vi "test_Import Configuration_Error.vi"(8 "error in (no error)":errorcluster, 11 "TestCase in":refnum<class "FPGA Addon Scripting API Unit Tests.lvclass">=refnum) -> (0 "error out":errorcluster, 3 "TestCase out":refnum<class "FPGA Addon Scripting API Unit Tests.lvclass">)   [LabVIEW 2026, in "FPGA Addon Scripting API Unit Tests.lvclass"]
uses:
  FPGA Addon Scripting API Unit Tests.lvclass
  FPGA Addon Test Class/FPGA Addon Test Class.lvclass
  APIs/Scripting API/Scripting API.lvlib
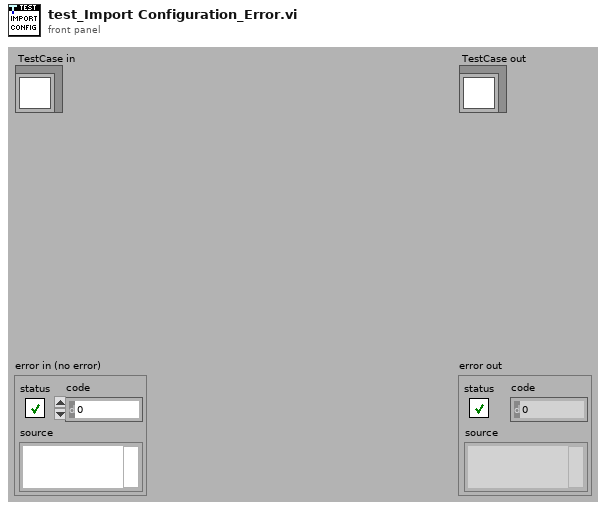
[diagram p1: front panel]
types:
  T1 = typedef "Custom Device API.lvlib/Custom Device Item Ref.ctl" = u64
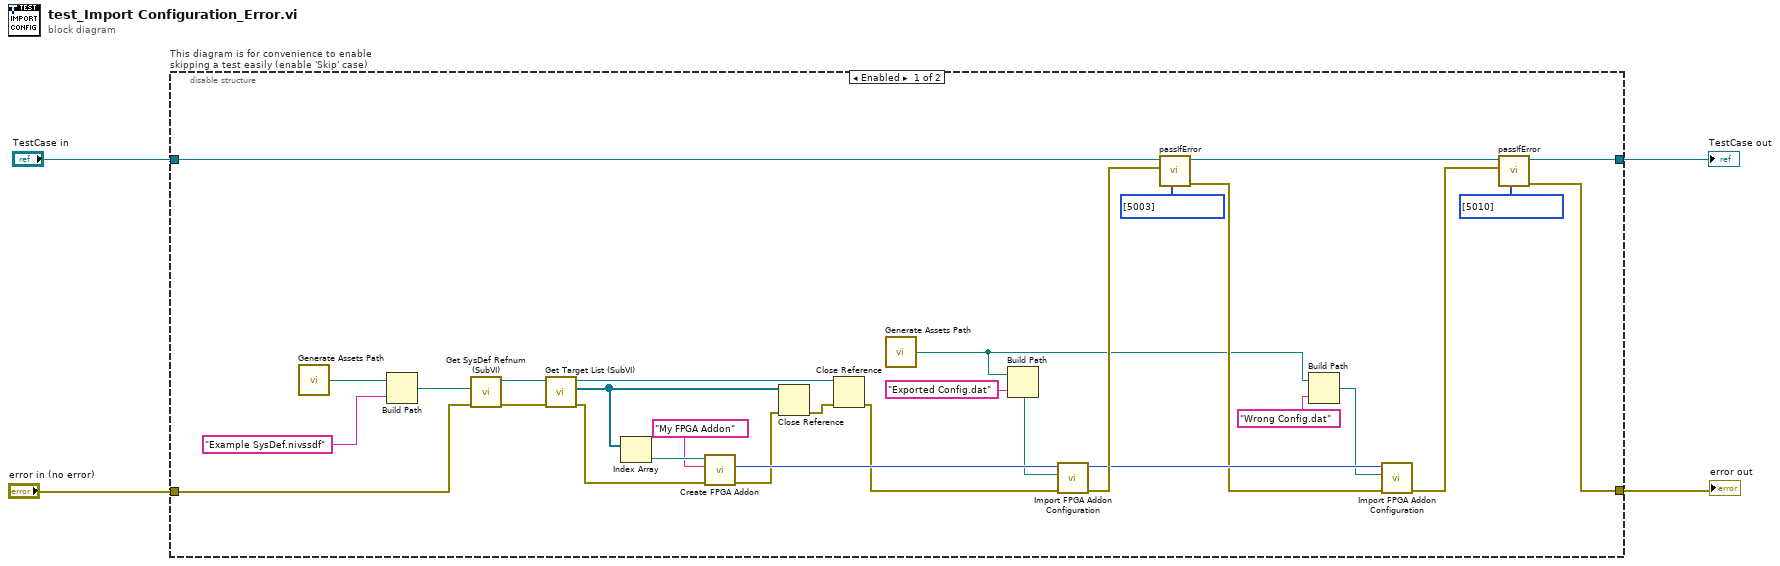
[diagram p0: block diagram]
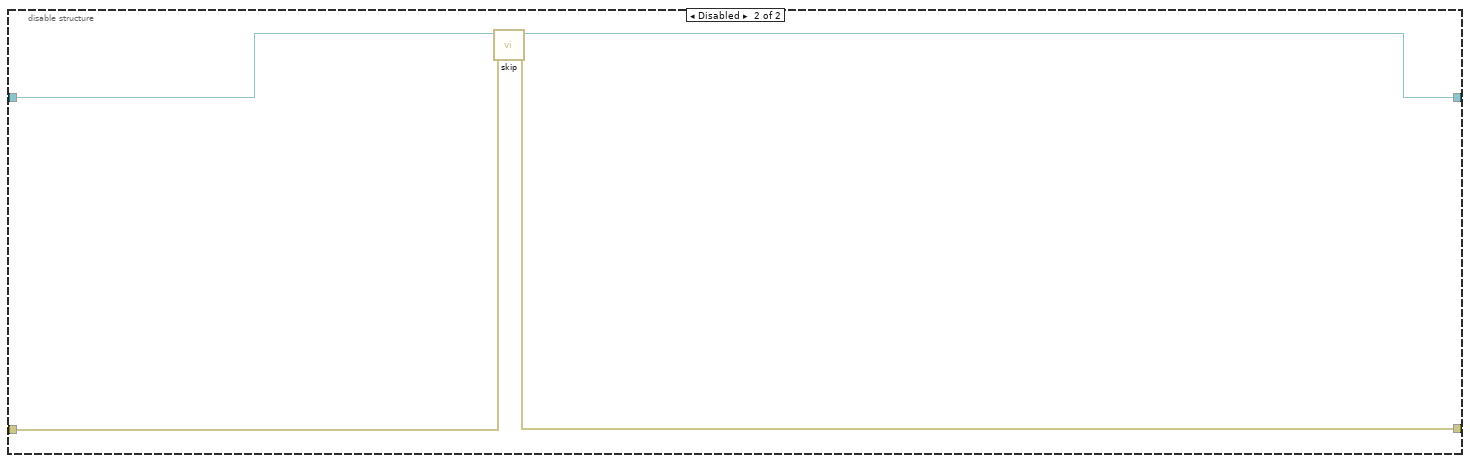
[diagram p2: hidden frame]
diagram:
  n1 = disable-structure "This diagram is for convenience to enable skipping a test easily (enable 'Skip' case)" shown="Enabled" {
    disable-tunnel: "TestCase in" -> [w17 w38]
    disable-tunnel: [w6 w36] -> w1
    disable-tunnel: [w5 w37] -> w3
    disable-tunnel: "error in (no error)" -> [w30 w35]
    frame Enabled {
      n2 = call "Generate Assets Path.vi"() -> ("Assets path"=w34:path)
      n3 = Build Path(base path=w34, name or relative path="Example SysDef.nivssdf") -> (appended path=w32:path)
      n4 = call "Get SysDef Refnum (SubVI).vi"("error in (no error)"=w30, "System Definition path"=w32) -> ("error out"=w29:errorcluster, "NationalInstruments.VeriStand.SystemDefinitionAPI.SystemDefinition"=w31:refnum<k39>)  [unwired: 8 in]
      n5 = call "Get Target List (SubVI).vi"("error in (no error)"=w29, "NationalInstruments.VeriStand.SystemDefinitionAPI.SystemDefinition"=w31) -> ("error out"=w28:errorcluster, "Target List Refnums"=w21:refnum<k39>[], "NationalInstruments.VeriStand.SystemDefinitionAPI.SystemDefinition"=w22:refnum<k39>)  [unwired: 7 in]
      n6 = Index Array(array=w21) -> (element=w27:refnum<k39>)  [unwired: 1 in]
      n7 = call "Create FPGA Addon.vi"("error in"=w28, "FPGA addon name"="My FPGA Addon", "NationalInstruments.VeriStand.SystemDefinitionAPI.Target"=w27) -> ("error out"=w20:errorcluster, "FPGA addon refnum"=w25:T1)  [unwired: 6 in, 1 out]
      n8 = Close Reference(reference=w21, error in (no error)=w20) -> (error out=w19:errorcluster)
      n9 = Close Reference(reference=w22, error in (no error)=w19) -> (error out=w18:errorcluster)
      n10 = call "Generate Assets Path.vi"() -> ("Assets path"=w12:path)
      n11 = Build Path(base path=w12, name or relative path="Exported Config.dat") -> (appended path=w23:path)
      n12 = call "Import FPGA Addon Configuration.vi"("error in"=w18, "configuration file path"=w23, "FPGA addon refnum in"=w25) -> ("error out"=w16:errorcluster, "FPGA addon refnum out"=w14:T1)  [unwired: 7 in]
      n13 = call-dynamic "passIfError.vi"("passing error codes (default = any error code)"=i32[] [5003], "error"=w16, "TestCase in"=w17) -> ("error out"=w13:errorcluster, "TestCase out"=w8:refnum<class "FPGA Addon Scripting API Unit Tests.lvclass">)  [unwired: 7 in]
      n14 = Build Path(base path=w12, name or relative path="Wrong Config.dat") -> (appended path=w10:path)
      n15 = call "Import FPGA Addon Configuration.vi"("error in"=w13, "configuration file path"=w10, "FPGA addon refnum in"=w14) -> ("error out"=w7:errorcluster)  [unwired: 7 in, 1 out]
      n16 = call-dynamic "passIfError.vi"("passing error codes (default = any error code)"=i32[] [5010], "error"=w7, "TestCase in"=w8) -> ("error out"=w5:errorcluster, "TestCase out"=w6:refnum<class "FPGA Addon Scripting API Unit Tests.lvclass">)  [unwired: 7 in]
    }
    frame Disabled {
      # "skip test result while test is under development"
      n17 = call <vilib>:"skip.vi"("error in (no error)"=w35, "TestCase in"=w38) -> ("error out"=w37:errorcluster, "TestCase out"=w36:refnum<class "FPGA Addon Scripting API Unit Tests.lvclass">)  [unwired: 8 in]
    }
  }
  "error out" <- w3
  "TestCase out" <- w1
